vi "Focus Configure.vi"(8 "error in (no error)":errorcluster, 11 "ArduinoFocus in":refnum<class "ArduinoFocus.lvclass">) -> (0 "error out":errorcluster, 3 "ArduinoFocus out":refnum<class "ArduinoFocus.lvclass">)   [LabVIEW 2022 SP3, in "ArduinoFocus.lvclass"]
uses:
  ArduinoFocus.lvclass
  ArduinoFocus.lvclass/ArduinoFocus.ctl
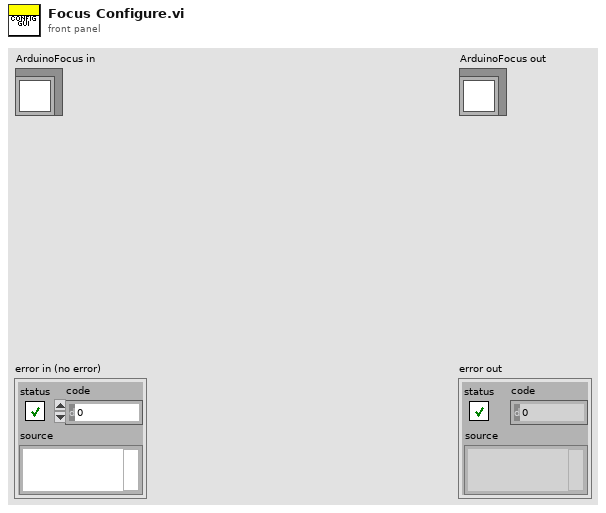
[diagram p1: front panel]
types:
  T1 = typedef "ArduinoFocus.lvclass/Arduino Focus cluster Settings.ctl" = cluster{"Port":refnum<visa-resource-name>, "Homing Parameters":T2, "Positions":i32[], "Homed":bool[]}
  T2 = typedef "arduino Motor Control cluster Command.ctl" = cluster{"Direction":bool, "NUMBER OF  STEPS":u32, "SPEED STEPS/SEC":u16, "ACC/DECEL STEPS/SEC^2":u16, "EN/DIS?":bool}
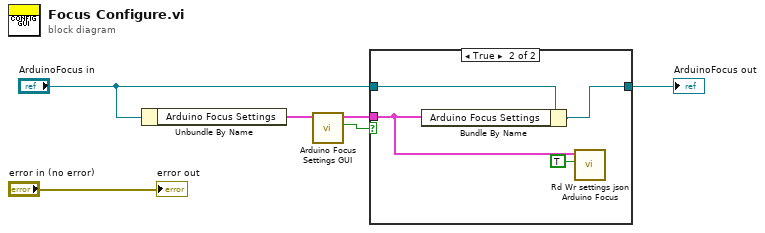
[diagram p0: block diagram]
diagram:
  n1 = Unbundle By Name("ArduinoFocus in") -> ("Arduino Focus Settings"=w5:T1)
  n2 = call "Arduino Focus Settings GUI.vi"("Arduino Focus Settings"=w5) -> ("Save?"=w4:bool, "Settings out"=w2:T1)  [unwired: 9 in]
  n3 = case shown="True" w4 {
    tunnel: "ArduinoFocus in" -> [w7 w11]
    tunnel: w2 -> [_ w10]
    tunnel: [w7 w8] -> w1
    frame False {
    }
    frame True {
      n4 = Bundle By Name(cluster=w11, "Arduino Focus Settings"=w10) -> (w8:refnum<class "ArduinoFocus.lvclass">)
      n5 = call "Rd Wr settings json Arduino Focus.vi"("Write? (F:Read)"=TRUE, "Arduino Focus Settings"=w10) -> ()  [unwired: 8 in, 2 out]
    }
  }
  "ArduinoFocus out" <- w1
  "error out" <- "error in (no error)"
